vi "Receive.vi"(7 "path override":path, 8 "error in (no error)":errorcluster, 9 "flags_":i32, 10 "buf in":string, 11 "s":u64) -> (0 "error out":errorcluster, 2 "buf out":string, 3 "s_":u64)   [LabVIEW 2025, in "LibZMQ.lvlib"]
uses:
  LibZMQ.lvlib
  errno.vi
  strerror.vi
  <vilib>/Utility/error.llb/Error Cluster From Error Code.vi
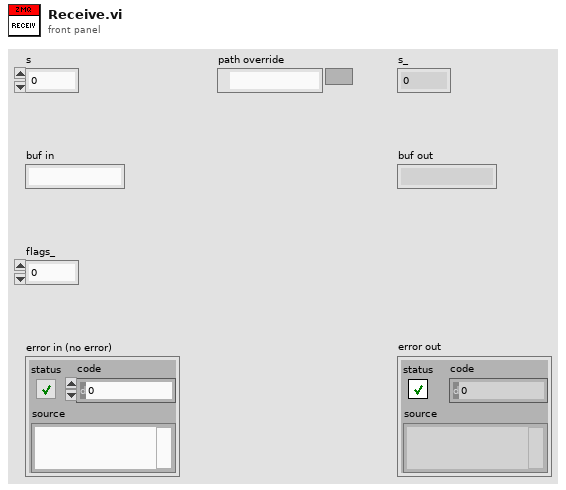
[diagram p1: front panel]
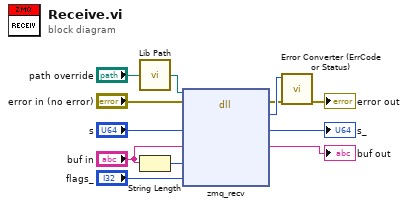
[diagram p0: block diagram]
diagram:
  n1 = call "Lib Path.vi"("path override"="path override") -> ("lib path"=w1:path)
  n2 = String Length(string="buf in") -> (length=w5:i32)
  n3 = dll-call lib="home/james/Documents/ZeroMQ_LV/libzmq-v143-mt-4_3_6/libzmq.so" fn="zmq_recv"(path in=w1, error in="error in (no error)", "s_"="s", "buf"="buf in", "len"=w5, "flags_"="flags_") -> (error out=w11:errorcluster, "return type"=w12:i32, "s_"=→"s_":u64, "buf"=→"buf out":string)  [unwired: 3 in, 1 out]
  n4 = call "Error Converter (ErrCode or Status).vi"("error in (no error)"=w11, "error code"=w12) -> ("error out"=→"error out":errorcluster)  [unwired: 9 in]
